vi "Refresh Controls.vi"(8 "error in":errorcluster, 11 "Electronic Load in":refnum<class "Electronic Load.lvclass">) -> (0 "error out":errorcluster, 3 "Electronic Load out":refnum<class "Electronic Load.lvclass">)   [LabVIEW 2019, in "Electronic Load.lvlib" / "Electronic Load.lvclass"]
uses:
  Library/Electronic Load.lvclass
  Library/Electronic Load.lvclass/Electronic Load.ctl
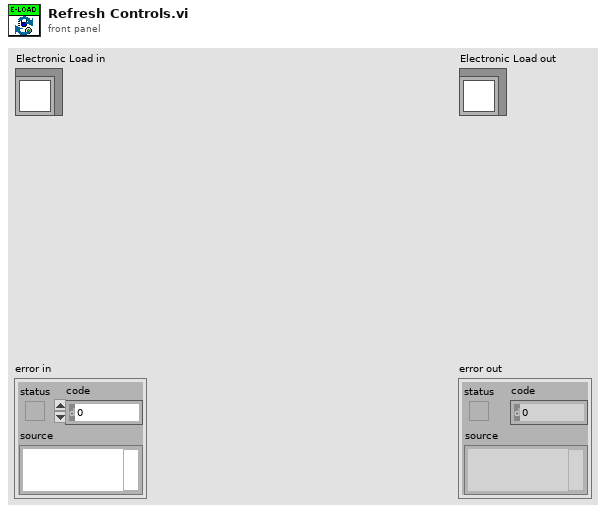
[diagram p1: front panel]
types:
  T1 = typedef "Electronic Load.lvlib/Electronic Load.lvclass/OCP Settings.ctl" = cluster{"OCP_Enabled":bool, "OCP Level":dbl, "OCP Delay":dbl}
  T2 = typedef "Electronic Load.lvlib/Electronic Load.lvclass/E-Load Function.ctl" = cluster{"Mode":T3, "Input Level":dbl, "Output":bool, "Slew Rate":dbl}
  T3 = typedef "Electronic Load.lvlib/Electronic Load.lvclass/E-Load Mode.ctl" = enum16{"Current", "Resistance", "Voltage"}
  T4 = typedef "Electronic Load.lvlib/Electronic Load.lvclass/Trigger Settings.ctl" = cluster{"Mode":T3, "Initial":dbl, "Transient":dbl, "Interval":dbl, "Width":dbl, "Delay":dbl, "Data Pts":i32, "Slew Rate":dbl}
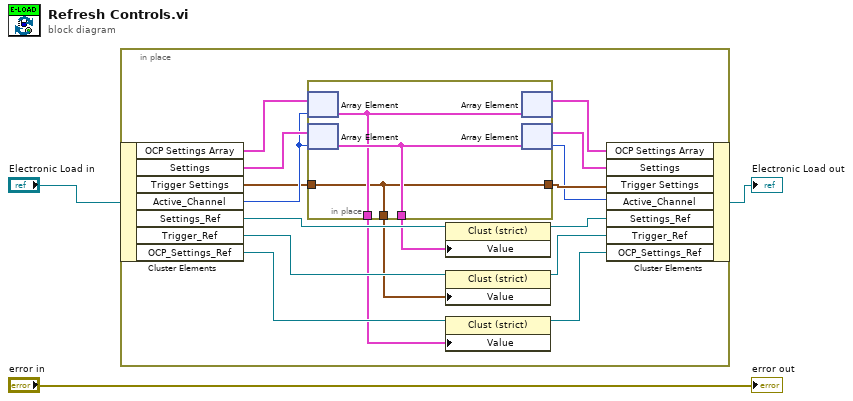
[diagram p0: block diagram]
diagram:
  n1 = in-place {
    n2 = in-place-cluster #1("Electronic Load in") -> ("OCP Settings Array"=w11:T1[], "Settings"=w20:T2[], "Trigger Settings"=w5:T4, "Active_Channel"=w10:u32, "Settings_Ref"=w18:refnum<vi>, "Trigger_Ref"=w16:refnum<vi>, "OCP_Settings_Ref"=w8:refnum<vi>)
    n3 = in-place {
      in-place-border: [w21] -> w14
      in-place-border: [w23] -> w13
      in-place-border: [w22] -> w7
      in-place-border: [w21] -> w6
      in-place-border: w5 -> [w21]
      n4 = in-place-array #2(w11, w10) -> (w22:T1)
      n5 = in-place-array #3(w20, w10) -> (w23:T2)
      n6 = in-place-array #2(w22) -> (w12:T1[])  [unwired: 1 out]
      n7 = in-place-array #3(w23) -> (w19:T2[], w4:i32)
    }
    n8 = property class="Clust (strict)"(reference=w18, "Value"=w13) -> (reference out=w17:refnum<vi>)  [unwired: 1 in, 1 out]
    n9 = property class="Clust (strict)"(reference=w16, "Value"=w14) -> (reference out=w15:refnum<vi>)  [unwired: 1 in, 1 out]
    n10 = property class="Clust (strict)"(reference=w8, "Value"=w7) -> (reference out=w9:refnum<vi>)  [unwired: 1 in, 1 out]
    n11 = in-place-cluster #1("OCP Settings Array"=w12, "Settings"=w19, "Trigger Settings"=w6, "Active_Channel"=w4, "Settings_Ref"=w17, "Trigger_Ref"=w15, "OCP_Settings_Ref"=w9) -> (→"Electronic Load out":refnum<class "Electronic Load.lvclass">)
  }
  "error out" <- "error in"
